vi "reprTextual.vi"(8 "error in (no error)":errorcluster, 11 "RoundBuoy in":refnum<class "RoundBuoy.lvclass">) -> (0 "error out":errorcluster, 2 "Description":string, 3 "RoundBuoy out":refnum<class "RoundBuoy.lvclass">)   [LabVIEW 2011, in "RoundBuoy.lvclass"]
uses:
  RoundBuoy.lvclass
  RoundBuoy.lvclass/RoundBuoy.ctl
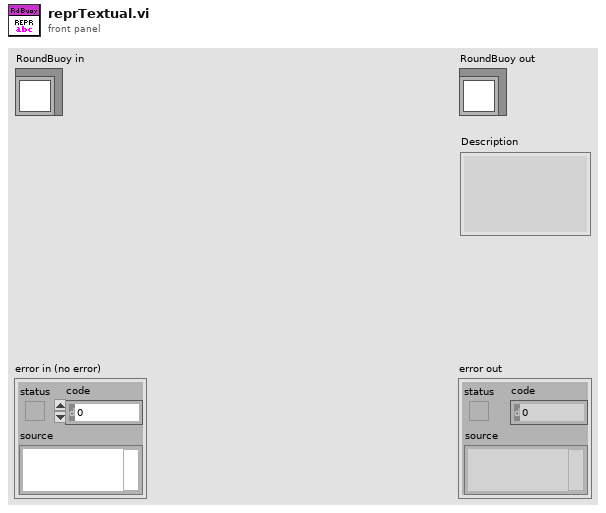
[diagram p1: front panel]
types:
  T1 = typedef "UTM Location.ctl" = cluster{"UTM Zone":dbl, "Hemisphere":enum16{"North", "South"}, "East":dbl, "North":dbl}
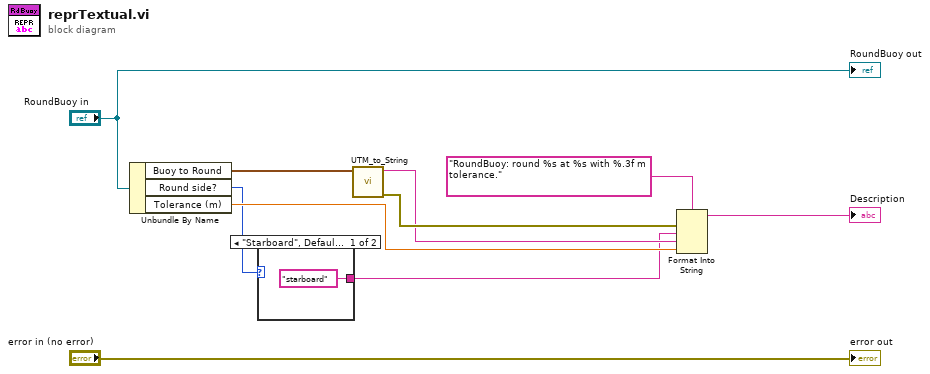
[diagram p0: block diagram]
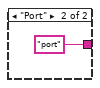
[diagram p2: hidden frame]
diagram:
  n1 = Unbundle By Name("RoundBuoy in") -> ("Buoy to Round"=w6:T1, "Round side?"=w3:enum16{"Starboard", "Port"}, "Tolerance (m)"=w4:dbl)
  n2 = case shown="\"Starboard\", Default" w3 {
    tunnel: ["starboard" ("UTM String") "port" ("UTM String")] -> w2
    frame "Starboard", Default {
    }
    frame "Port" {
    }
  }
  n3 = call "UTM_to_String.vi"("UTM Location"=w6) -> ("error out"=w8:errorcluster, "UTM String"=w5:string)  [unwired: 9 in]
  n4 = Format Into String(format string="RoundBuoy: round %s at %s with %.3f m tolerance.", error in=w8, w2, w5, w4) -> (resulting string=→"Description":string)  [unwired: 1 in, 1 out]
  "error out" <- "error in (no error)"
  "RoundBuoy out" <- "RoundBuoy in"
